vi "Close Refnum.vi"(8 "Error In":errorcluster, 11 "NumericOperation in":refnum<class "NumericOperation.lvclass">) -> (0 "Error Out":errorcluster, 3 "NumericOperation out":refnum<class "NumericOperation.lvclass">)   [LabVIEW 2021, in "Calculator.lvlib" / "NumericOperation.lvclass"]
doc: "This VI is an overriding method which overrides to its child classes based on the object wired and closes the subpanel reference."
uses:
  NumericOperation.lvclass
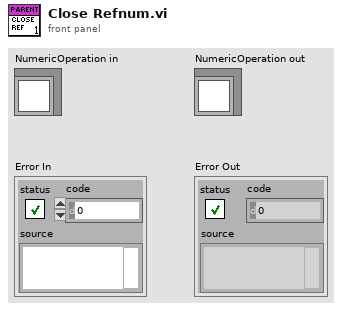
[diagram p1: front panel]
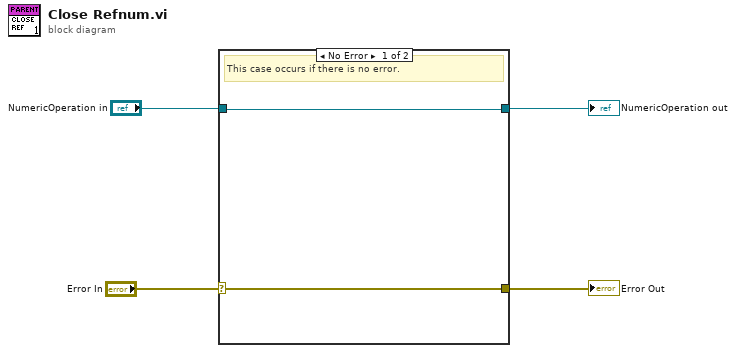
[diagram p0: block diagram]
diagram:
  n1 = case shown="No Error" "Error In" {
    selector: "Error In" -> [w5 w8]
    tunnel: [w5 w8] -> w3
    tunnel: [w6 w7] -> w1
    tunnel: "NumericOperation in" -> [w6 w7]
    frame No Error {
      # "This case occurs if there is no error."
    }
    frame Error {
      # "This case occurs if there is any error."
    }
  }
  "Error Out" <- w3
  "NumericOperation out" <- w1
